vi "GridEye.vi"() -> ()   [LabVIEW 2011]
uses:
  <vilib>/gmath/interp.llb/Interpolate 2D (1d X,Y).vi
  <vilib>/gmath/NI_Gmath.lvlib
panel:
  in  "View Mode":u16(ring) items=["Back", "Front"]
  in  "temperature scaling":dbl=1.0 caption="x" format="%_4f"
  in  "?":T1(tab)
  out "Values 0":dbl[](array[numeric]) format="%.2g"
  out "Values 3":dbl[](array[numeric]) format="%.2g"
  out "Values 2":dbl[](array[numeric]) format="%.2g"
  out "Values 1":dbl[](array[numeric]) format="%.2g"
  out "Values 7":dbl[](array[numeric]) format="%.2g"
  out "Values 6":dbl[](array[numeric]) format="%.2g"
  out "Values 5":dbl[](array[numeric]) format="%.2g"
  out "Values 4":dbl[](array[numeric]) format="%.2g"
  out "temperature values":dbl[][](graph)=[[-24.0, -22.0, -20.0, -18.0, -16.0, -14.0, -12.0, -10.0], [-8.0, -6.0, -4.0, -2.0, 0.0, 2.0, 4.0, 6.0], [8.0, 10.0, 12.0, 14.0, 16.0, 18.0, 20.0, 22.0], [24.0, 26.0, 28.0, 30.0, 32.0, 34.0, 36.0, 38.0], [40.0, 42.0, 44.0, 46.0, 48.0, 50.0, 52.0, 54.0], [56.0, 58.0, 60.0, 62.0, 64.0, 66.0, 68.0, 70.0], [72.0, 74.0, 76.0, 78.0, 80.0, 82.0, 84.0, 86.0], [88.0, 90.0, 92.0, 94.0, 96.0, 98.0, 100.0, 102.0]]
  in  "Interpolation\nloops":u8(slide)=2 max=5 step=1 scale=0.0..5.0
  out "interpolated view":dbl[][](graph)=[[-24.0, -22.0, -20.0, -18.0, -16.0, -14.0, -12.0, -10.0], [-8.0, -6.0, -4.0, -2.0, 0.0, 2.0, 4.0, 6.0], [8.0, 10.0, 12.0, 14.0, 16.0, 18.0, 20.0, 22.0], [24.0, 26.0, 28.0, 30.0, 32.0, 34.0, 36.0, 38.0], [40.0, 42.0, 44.0, 46.0, 48.0, 50.0, 52.0, 54.0], [56.0, 58.0, 60.0, 62.0, 64.0, 66.0, 68.0, 70.0], [72.0, 74.0, 76.0, 78.0, 80.0, 82.0, 84.0, 86.0], [88.0, 90.0, 92.0, 94.0, 96.0, 98.0, 100.0, 102.0]]
  out "Thermistor temperature":dbl caption="°C" format="%.4g"
  in  "temperature to color scaling":enum32{"manual", "automatic"}(tab)
  in  "max":dbl=100.0 caption="°C"
  in  "min":dbl=-20.0 caption="°C"
  in  "Auto scale step size":u8=1 caption="°C"
  in  "Spread spectrum":bool
  in  "Update Speed":u16(ring) items=["10 Hz", "1 Hz"]
  in  "Output Mode":u16(ring) items=["normal", "moving average"]
  # "Enables a better visualization\nof temperature differences"
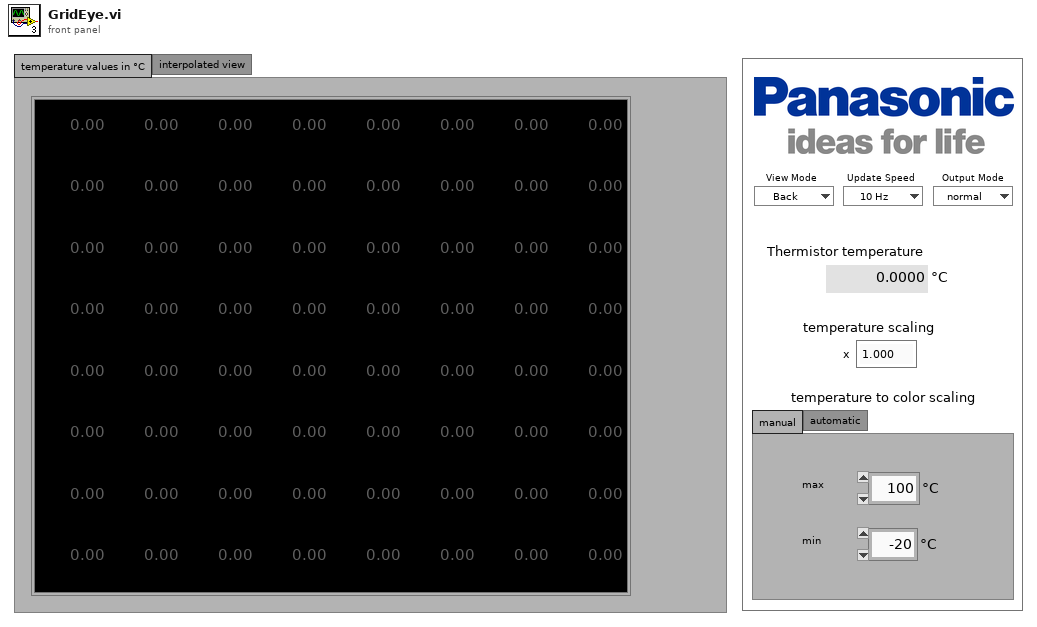
[diagram p1: front panel]
types:
  T1 = enum32{"temperature values in °C", "interpolated view"}
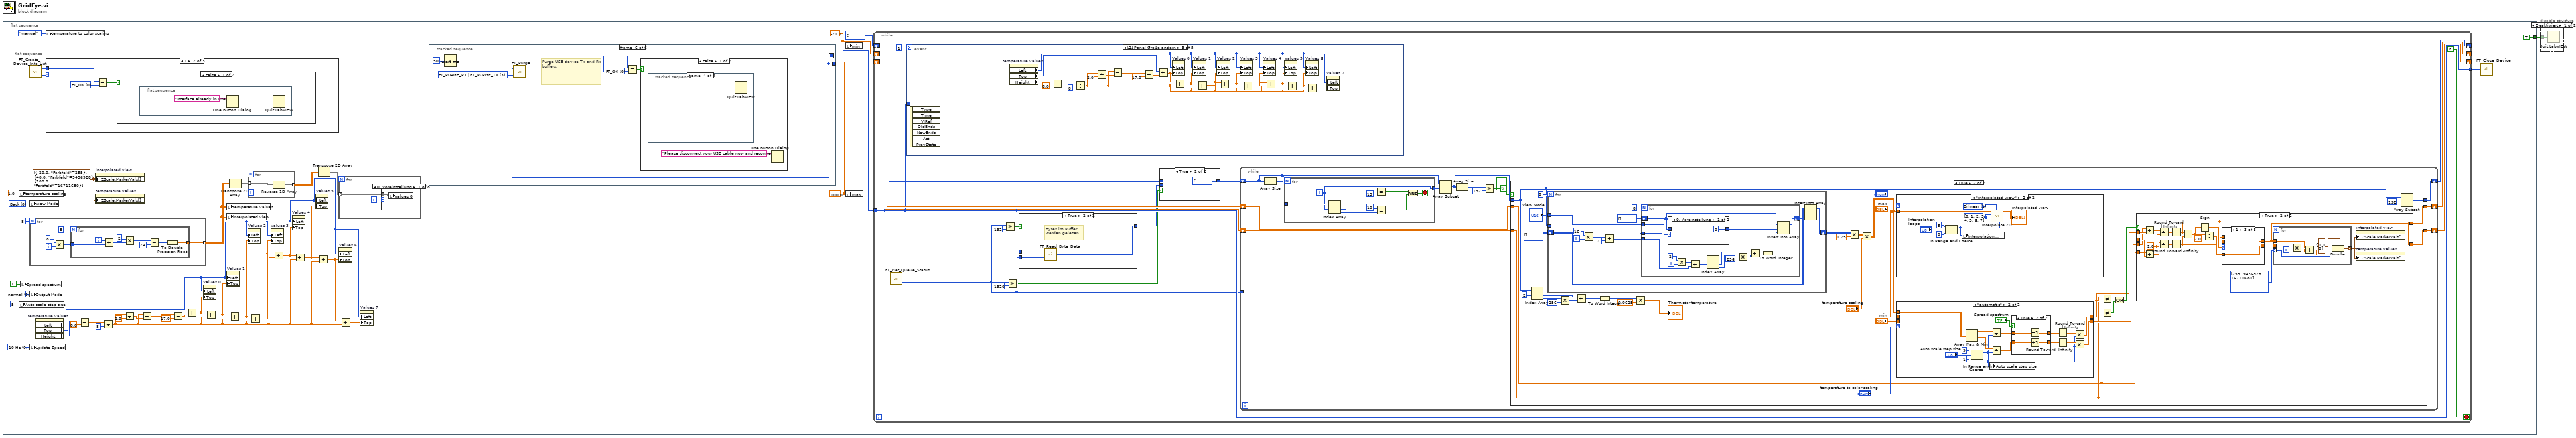
[diagram p0: block diagram]
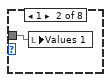
[diagram p3: hidden frame]
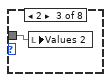
[diagram p4: hidden frame]
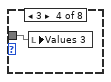
[diagram p5: hidden frame]
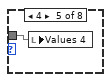
[diagram p6: hidden frame]
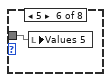
[diagram p7: hidden frame]
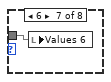
[diagram p8: hidden frame]
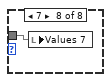
[diagram p9: hidden frame]
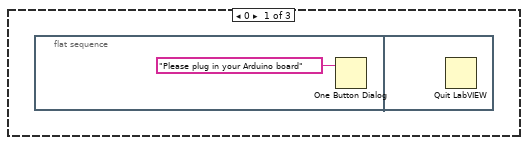
[diagram p10: hidden frame]
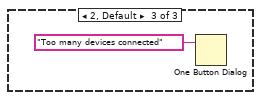
[diagram p12: hidden frame]
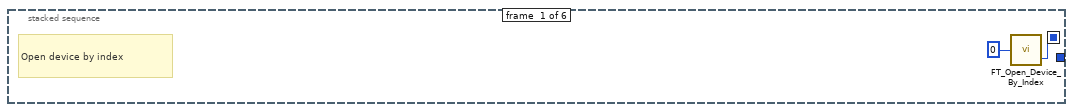
[diagram p13: hidden frame]
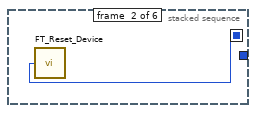
[diagram p14: hidden frame]
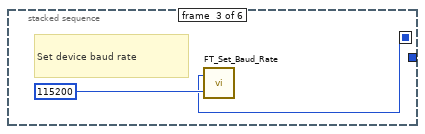
[diagram p15: hidden frame]
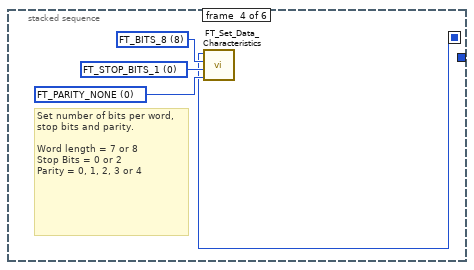
[diagram p16: hidden frame]
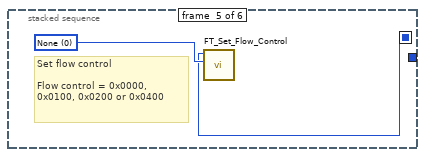
[diagram p17: hidden frame]
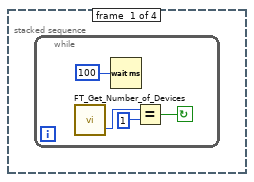
[diagram p18: hidden frame]
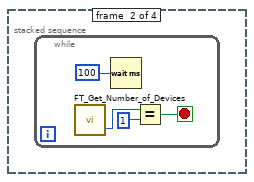
[diagram p19: hidden frame]
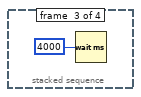
[diagram p20: hidden frame]
diagram:
  n1 = flat-sequence {
    tunnel: [TRUE ("Stopp? (T)")] -> w1
    frame #0 {
      w22 = u16 0 items=["Back", "Front"] ("View Mode")
      w25 = cluster{dbl, "Farbfeld":u32}[] [{-20.0, "Farbfeld"=255}, {40.0, "Farbfeld"=9436928}, {100.0, "Farbfeld"=16711680}] ("Array")
      w33 = u16 0 items=["normal", "moving average"] ("Output Mode")
      w34 = u16 0 items=["10 Hz", "1 Hz"] ("Update Speed")
      n2 = flat-sequence {
        frame #0 {
          n3 = call "FT_Create_Device_Info_List.vi"() -> ("Number of Devices"=w45:u32, "FT_Status"=w46:u32)
          n4 = case shown="1" w45 {
            tunnel: w46 -> [_ w50 _]
            frame 0 {
              n5 = flat-sequence {
                frame #0 {
                  n6 = One Button Dialog(message="Please plug in your Arduino board" ("Nachricht")) -> ()  [unwired: 1 in, 1 out]
                }
                frame #1 {
                  n7 = Quit LabVIEW() -> ()  [unwired: 1 in]
                }
              }
            }
            frame 1 {
              w49 = u32 0 items=["FT_OK", "FT_INVALID_HANDLE", "FT_DEVICE_NOT_FOUND", "FT_DEVICE_NOT_OPENED", "FT_IO_ERROR", "FT_INSUFFICIENT_RESOURCES", "FT_INVALID_PARAMETER", "FT_INVALID_BAUD_RATE", "FT_DEVICE_NOT_OPENED_FOR_ERASE", "FT_DEVICE_NOT_OPENED_FOR_WRITE", "FT_FAILED_TO_WRITE_DEVICE", "FT_EEPROM_READ_FAILED", "FT_EEPROM_WRITE_FAILED", "FT_EEPROM_ERASE_FAILED", "FT_EEPROM_NOT_PRESENT", "FT_EEPROM_NOT_PROGRAMMED", "FT_INVALID_ARGS", "FT_NOT_SUPPORTED", "FT_OTHER_ERROR"] ("FT_Status 4")
              n8 = Equal?(x=w50, y=w49) -> (x = y?=w48:bool)
              n9 = case shown="False" w48 {
                frame False {
                  n10 = flat-sequence {
                    frame #0 {
                      n11 = One Button Dialog(message="Interface already in use" ("Nachricht")) -> ()  [unwired: 1 in, 1 out]
                    }
                    frame #1 {
                      n12 = Quit LabVIEW() -> ()  [unwired: 1 in]
                    }
                  }
                }
                frame True {
                }
              }
            }
            frame 2, Default {
              n13 = One Button Dialog(message="Too many devices connected" ("Nachricht")) -> ()  [unwired: 1 in, 1 out]
            }
          }
        }
      }
      n14 = local write "temperature scaling"(1.0 ("temperature scaling")) -> ()
      n15 = local write "Auto scale step size"(u8 5 ("Autoscale step size")) -> ()
      n16 = local write "Spread spectrum"(TRUE ("stop")) -> ()
      n17 = local write "View Mode"(w22) -> ()
      n18 = for {
        N: 8 -> [_]
        tunnel: [w55] -> w29 mode=indexing
        i -> [w58]
        n19 = Multiply(x=8, y=w58) -> (x*y=w56:i32)
        n20 = for {
          N: 8 -> [_]
          tunnel: w56 -> [w62]
          tunnel: [w60] -> w55 mode=indexing
          i -> [w64]
          n21 = Add(x=w64, y=w62) -> (x+y=w63:i32)
          n22 = Multiply(x=2, y=w63) -> (x*y=w65:i32)
          n23 = Subtract(x=w65, y=24) -> (x-y=w61:i32)
          n24 = To Double Precision Float(number=w61) -> (double precision float=w60:dbl)
        }
      }
      n25 = local write "Output Mode"(w33) -> ()
      n26 = local write "Update Speed"(w34) -> ()
      n27 = property on="temperature values" class="IntGraph (strikt)"() -> ("Left"=w4:i32, "Top"=w3:i32, "Height"=w2:u32)  [unwired: 2 in, 2 out]
      n28 = local write "temperature to color scaling"(enum32{"manual", "automatic"}."manual" ("temperature to color scaling")) -> ()
      n29 = Subtract(x=w2, y=8.0) -> (x-y=w21:dbl)
      n30 = property on="interpolated view" class="IntGraph (strikt)"("ZScale.MarkerVals[]"=w25) -> ()  [unwired: 2 in, 2 out]
      n31 = property on="temperature values" class="IntGraph (strikt)"("ZScale.MarkerVals[]"=w25) -> ()  [unwired: 2 in, 2 out]
      n32 = Divide(x=w21, y=u32 8) -> (x/y=w19:dbl)
      n33 = Divide(x=w19, y=2.0) -> (x/y=w15:dbl)
      n34 = Subtract(x=w19, y=w15) -> (x-y=w16:dbl)
      n35 = Subtract(x=w16, y=17.0) -> (x-y=w18:dbl)
      n36 = Add(x=w3, y=w18) -> (x+y=w5:dbl)
      n37 = property on="Values 0" class="Arr (strikt)"("Left"=w4, "Top"=w5) -> ()  [unwired: 2 in, 2 out]
      n38 = Add(x=w5, y=w19) -> (x+y=w6:dbl)
      n39 = local write "temperature values"(w29) -> ()
      n40 = local write "interpolated view"(w29) -> ()
      n41 = property on="Values 1" class="Arr (strikt)"("Left"=w4, "Top"=w6) -> ()  [unwired: 2 in, 2 out]
      n42 = Add(x=w6, y=w19) -> (x+y=w7:dbl)
      n43 = Transpose 2D Array(2D array=w29) -> (transposed array=w31:dbl[][])
      n44 = for {
        tunnel: w31 -> [w54] mode=indexing
        tunnel: [w53] -> w30 mode=indexing
        n45 = Reverse 1D Array(array=w54) -> (reversed array=w53:dbl[])
      }
      n46 = property on="Values 2" class="Arr (strikt)"("Left"=w4, "Top"=w7) -> ()  [unwired: 2 in, 2 out]
      n47 = Add(x=w7, y=w19) -> (x+y=w8:dbl)
      n48 = property on="Values 3" class="Arr (strikt)"("Left"=w4, "Top"=w8) -> ()  [unwired: 2 in, 2 out]
      n49 = Add(x=w8, y=w19) -> (x+y=w9:dbl)
      n50 = property on="Values 4" class="Arr (strikt)"("Left"=w4, "Top"=w9) -> ()  [unwired: 2 in, 2 out]
      n51 = Add(x=w9, y=w19) -> (x+y=w10:dbl)
      n52 = property on="Values 5" class="Arr (strikt)"("Left"=w4, "Top"=w10) -> ()  [unwired: 2 in, 2 out]
      n53 = Add(x=w10, y=w19) -> (x+y=w11:dbl)
      n54 = Transpose 2D Array(2D array=w30) -> (transposed array=w28:dbl[][])
      n55 = for {
        tunnel: w28 -> [w35] mode=indexing
        i -> [w36]
        n56 = case shown="0, Voreinstellung" w36 {
          tunnel: w35 -> [w37 w38 w39 w40 w41 w42 w43 w44]
          frame 0, Default {
            n57 = local write "Values 0"(w37) -> ()
          }
          frame 1 {
            n58 = local write "Values 1"(w38) -> ()
          }
          frame 2 {
            n59 = local write "Values 2"(w39) -> ()
          }
          frame 3 {
            n60 = local write "Values 3"(w40) -> ()
          }
          frame 4 {
            n61 = local write "Values 4"(w41) -> ()
          }
          frame 5 {
            n62 = local write "Values 5"(w42) -> ()
          }
          frame 6 {
            n63 = local write "Values 6"(w43) -> ()
          }
          frame 7 {
            n64 = local write "Values 7"(w44) -> ()
          }
        }
      }
      n65 = property on="Values 6" class="Arr (strikt)"("Left"=w4, "Top"=w11) -> ()  [unwired: 2 in, 2 out]
      n66 = Add(x=w11, y=w19) -> (x+y=w12:dbl)
      n67 = property on="Values 7" class="Arr (strikt)"("Left"=w4, "Top"=w12) -> ()  [unwired: 2 in, 2 out]
    }
    frame #1 {
      w68 = -20.0 ("min")
      w69 = 100.0 ("max")
      n68 = stacked-sequence {
        seq-local: [w74 _ _ _ _ _] -> [_ w76 w77 w79 w83 w88]
        tunnel: [_ _ _ _ _ w88] -> w71
        frame #0 {
          # "Open device by index"
          n69 = call "FT_Open_Device_By_Index.vi"("Device Index"=u32 0) -> ("Handle"=w74:u32)  [unwired: 1 out]
        }
        frame #1 {
          n70 = call "FT_Reset_Device.vi"("Handle"=w76) -> ()  [unwired: 1 out]
        }
        frame #2 {
          # "Set device baud rate"
          n71 = call "FT_Set_Baud_Rate.vi"("Baud Rate"=u32 115200, "Handle"=w77) -> ()  [unwired: 1 out]
        }
        frame #3 {
          w81 = u8 0 items=["FT_PARITY_NONE", "FT_PARITY_ODD", "FT_PARITY_EVEN", "FT_PARITY_MARK", "FT_PARITY_SPACE"] ("Parity")
          w82 = u8 0 items=["FT_STOP_BITS_1"=0, "FT_STOP_BITS_2"=2] ("Stop Bits")
          w80 = u8 8 items=["FT_BITS_7"=7, "FT_BITS_8"=8] ("Word Length")
          # "Set number of bits per word, stop bits and parity.\n\nWord length = 7 or 8\nStop Bits = 0 or 2\nParity = 0, 1, 2, 3 or 4"
          n72 = call "FT_Set_Data_Characteristics.vi"("Parity"=w81, "Stop Bits"=w82, "Word Length"=w80, "Handle"=w79) -> ()  [unwired: 1 out]
        }
        frame #4 {
          w84 = u16 0 items=["None"=0, "RTS-CTS"=256, "DTR-DSR"=512, "XOn-XOff"=1024] ("Flow Control")
          # "Set flow control\n\nFlow control = 0x0000, 0x0100, 0x0200 or 0x0400"
          n73 = call "FT_Set_Flow_Control.vi"("Flow Control"=w84, "Handle"=w83) -> ()  [unwired: 2 in, 1 out]
        }
        frame #5 {
          w86 = u32 0 items=["FT_OK", "FT_INVALID_HANDLE", "FT_DEVICE_NOT_FOUND", "FT_DEVICE_NOT_OPENED", "FT_IO_ERROR", "FT_INSUFFICIENT_RESOURCES", "FT_INVALID_PARAMETER", "FT_INVALID_BAUD_RATE", "FT_DEVICE_NOT_OPENED_FOR_ERASE", "FT_DEVICE_NOT_OPENED_FOR_WRITE", "FT_FAILED_TO_WRITE_DEVICE", "FT_EEPROM_READ_FAILED", "FT_EEPROM_WRITE_FAILED", "FT_EEPROM_ERASE_FAILED", "FT_EEPROM_NOT_PRESENT", "FT_EEPROM_NOT_PROGRAMMED", "FT_INVALID_ARGS", "FT_NOT_SUPPORTED", "FT_OTHER_ERROR"] ("FT_Status 4")
          w90 = u32 3 items=["FT_PURGE_RX"=1, "FT_PURGE_TX"=2, "FT_PURGE_RX | FT_PURGE_TX"=3] ("Purge Flags")
          # "Purge USB device Tx and Rx  buffers."
          n74 = Wait (ms)(milliseconds to wait=u32 50 ("Zu wartende ms")) -> ()  [unwired: 1 out]
          n75 = call "FT_Purge.vi"("Purge Flags"=w90, "Handle"=w88) -> ("FT_Status"=w85:u32)
          n76 = Equal?(x=w85, y=w86) -> (x = y?=w87:bool)
          n77 = case shown="False" w87 {
            frame False {
              n78 = stacked-sequence {
                frame #0 {
                  n79 = while {
                    stop <- w94 continue-if-true
                    n80 = call "FT_Get_Number_of_Devices.vi"() -> ("Number of Devices"=w93:u16)  [unwired: 1 out]
                    n81 = Wait (ms)(milliseconds to wait=u32 100 ("Zu wartende ms")) -> ()  [unwired: 1 out]
                    n82 = Equal?(x=w93, y=u16 1) -> (x = y?=w94:bool)
                  }
                }
                frame #1 {
                  n83 = while {
                    stop <- w98 stop-if-true
                    n84 = call "FT_Get_Number_of_Devices.vi"() -> ("Number of Devices"=w97:u16)  [unwired: 1 out]
                    n85 = Wait (ms)(milliseconds to wait=u32 100 ("Zu wartende ms")) -> ()  [unwired: 1 out]
                    n86 = Equal?(x=w97, y=u16 1) -> (x = y?=w98:bool)
                  }
                }
                frame #2 {
                  n87 = Wait (ms)(milliseconds to wait=u32 4000 ("Zu wartende ms")) -> ()  [unwired: 1 out]
                }
                frame #3 {
                  n88 = Quit LabVIEW() -> ()  [unwired: 1 in]
                }
              }
              n89 = One Button Dialog(message="Please disconnect your USB cable now and reconnect it") -> ()  [unwired: 1 in, 1 out]
            }
            frame True {
            }
          }
        }
      }
      n90 = local write "min"(w68) -> ()
      n91 = local write "max"(w69) -> ()
      n92 = while {
        shift-right: [w116] -> _
        shift-left: u8[] [] -> [w104]
        tunnel: w71 -> [w110]
        tunnel: [w110] -> w70
        shift-right: [w113] -> _
        shift-left: w68 -> [w112]
        shift-right: [w109] -> _
        shift-left: w69 -> [w108]
        stop <- FALSE stop-if-true
        n93 = call "FT_Get_Queue_Status.vi"("Handle"=w110) -> ("Bytes Waiting"=w106:u32)  [unwired: 1 out]
        n94 = event shown="[2] Panel-Größe ändern" {
          selector: _ -> [_ _ _ _ _]
          dyn-events: _ -> [_ _ _ _ _]
          timeout: 1 -> [_ _ _ _ _]
          tunnel: w110 -> [_ w121 _ w147 w155]
          event Timeout {
            n95 = event-data() -> ()  [unwired: 1 in, 2 out]
          }
          event "Update Speed": Value Change {
            n96 = event-data() -> ("NewVal"=w125:u16)  [unwired: 1 in, 4 out]
            n97 = Build Array(u16 2 ("NeuerWert"), w125) -> (w122:u16[])
            n98 = Array Size(array=w122) -> (size(s)=w124:i32)
            n99 = To Unsigned Long Integer(number=w124) -> (unsigned 32bit integer=w123:u32)
            n100 = call "FT_Write_Byte_Data.vi"("Bytes To Write"=w123, "Buffer"=w122, "Handle"=w121) -> ()  [unwired: 2 out]
          }
          event Panel Resize {
            n101 = event-data() -> ()  [unwired: 1 in, 7 out]
            n102 = property on="temperature values" class="IntGraph (strikt)"() -> ("Left"=w133:i32, "Top"=w140:i32, "Height"=w128:u32)  [unwired: 2 in, 2 out]
            n103 = Subtract(x=w128, y=8.0) -> (x-y=w127:dbl)
            n104 = Divide(x=w127, y=u32 8) -> (x/y=w131:dbl)
            n105 = Divide(x=w131, y=2.0) -> (x/y=w144:dbl)
            n106 = Subtract(x=w131, y=w144) -> (x-y=w143:dbl)
            n107 = Subtract(x=w143, y=17.0) -> (x-y=w141:dbl)
            n108 = Add(x=w140, y=w141) -> (x+y=w139:dbl)
            n109 = property on="Values 0" class="Arr (strikt)"("Left"=w133, "Top"=w139) -> ()  [unwired: 2 in, 2 out]
            n110 = Add(x=w139, y=w131) -> (x+y=w138:dbl)
            n111 = property on="Values 1" class="Arr (strikt)"("Left"=w133, "Top"=w138) -> ()  [unwired: 2 in, 2 out]
            n112 = Add(x=w138, y=w131) -> (x+y=w137:dbl)
            n113 = property on="Values 2" class="Arr (strikt)"("Left"=w133, "Top"=w137) -> ()  [unwired: 2 in, 2 out]
            n114 = Add(x=w137, y=w131) -> (x+y=w136:dbl)
            n115 = property on="Values 3" class="Arr (strikt)"("Left"=w133, "Top"=w136) -> ()  [unwired: 2 in, 2 out]
            n116 = Add(x=w136, y=w131) -> (x+y=w135:dbl)
            n117 = property on="Values 4" class="Arr (strikt)"("Left"=w133, "Top"=w135) -> ()  [unwired: 2 in, 2 out]
            n118 = Add(x=w135, y=w131) -> (x+y=w134:dbl)
            n119 = property on="Values 5" class="Arr (strikt)"("Left"=w133, "Top"=w134) -> ()  [unwired: 2 in, 2 out]
            n120 = Add(x=w134, y=w131) -> (x+y=w132:dbl)
            n121 = property on="Values 6" class="Arr (strikt)"("Left"=w133, "Top"=w132) -> ()  [unwired: 2 in, 2 out]
            n122 = Add(x=w132, y=w131) -> (x+y=w130:dbl)
            n123 = property on="Values 7" class="Arr (strikt)"("Left"=w133, "Top"=w130) -> ()  [unwired: 2 in, 2 out]
          }
          event "Output Mode": Value Change {
            n124 = event-data() -> ("NewVal"=w153:u16)  [unwired: 1 in, 4 out]
            n125 = Scale By Power Of 2(n=5, x=w153) -> (x*2^n=w151:u16)
            n126 = Build Array(u16 7 ("NeuerWert"), w151) -> (w148:u16[])
            n127 = Array Size(array=w148) -> (size(s)=w150:i32)
            n128 = To Unsigned Long Integer(number=w150) -> (unsigned 32bit integer=w149:u32)
            n129 = call "FT_Write_Byte_Data.vi"("Bytes To Write"=w149, "Buffer"=w148, "Handle"=w147) -> ()  [unwired: 2 out]
          }
          event Application Instance Close? {
            n130 = event-data() -> ("SilentShutdown"=w156:bool)  [unwired: 1 in, 3 out]
            n131 = call "FT_Close_Device.vi"("Handle"=w155) -> ()  [unwired: 1 out]
            n132 = event-data("SilentShutdown"=w156) -> ()  [unwired: 2 in, 1 out]
          }
        }
        n133 = Greater Or Equal?(x=w106, y=u32 132) -> (x >= y?=w114:bool)
        n134 = Greater Or Equal?(x=w106, y=u32 1320) -> (x >= y?=w105:bool)
        n135 = case shown="True" w114 {
          tunnel: [u8[] [] ("Read Data") w160] -> w102
          tunnel: w110 -> [_ w158]
          tunnel: w106 -> [_ w159]
          frame False {
          }
          frame True {
            # "Bytes im Puffer werden gelesen."
            n136 = call "FT_Read_Byte_Data.vi"("Handle"=w158, "Bytes To Read"=w159) -> ("Read Data"=w160:u8[])  [unwired: 2 out]
          }
        }
        n137 = case shown="True" w105 {
          tunnel: w104 -> [w119 _]
          tunnel: [w118 u8[] []] -> w103
          tunnel: w102 -> [w117 _]
          frame False {
            n138 = Insert Into Array(array=w119, new element=w117) -> (w118:u8[])  [unwired: 1 in]
          }
          frame True {
          }
        }
        n139 = while {
          shift-right: [w166] -> w116
          shift-left: w103 -> [w172]
          tunnel: w106 -> [_]
          shift-right: [w164] -> w113
          shift-left: w112 -> [w163]
          shift-right: [w162] -> w109
          shift-left: w108 -> [w161]
          stop <- w167 continue-if-true
          n140 = Array Size(array=w172) -> (size(s)=w171:i32)
          n141 = for {
            N: w171 -> [_]
            tunnel: w172 -> [w327]
            tunnel: [w325] -> w165
            i -> [w325]
            stop <- w326 stop-if-true
            n142 = Index Array(array=w327, index #1=w325) -> (element #1=w328:u8, element #2=w330:u8)  [unwired: 1 in]
            n143 = Equal?(x=w328, y=u8 13) -> (x = y?=w331:bool)
            n144 = Equal?(x=u8 10 ("y"), y=w330) -> (x = y?=w332:bool)
            n145 = And(x=w331, y=w332) -> (x .and. y?=w326:bool)
          }
          n146 = Array Subset(array=w172, index=w165) -> (w168:u8[])  [unwired: 1 in]
          n147 = Array Size(array=w168) -> (size(s)=w170:i32)
          n148 = Greater Or Equal?(x=w170, y=132) -> (x >= y?=w167:bool)
          n149 = case shown="True" w167 {
            tunnel: w168 -> [w175 w192]
            tunnel: [w175 w206] -> w166
            tunnel: [w174 w183] -> w164
            tunnel: w163 -> [w174 w185]
            tunnel: [w173 w182] -> w162
            tunnel: w161 -> [w173 w184]
            frame False {
            }
            frame True {
              n150 = Index Array(array=w192, index #1=2 ("Index")) -> (element #1=w199:u8, element #2=w200:u8)  [unwired: 1 in]
              n151 = for {
                N: 8 -> [_]
                tunnel: w192 -> [w304]
                shift-right: [w295] -> w178
                shift-left: i16[][] [] -> [w297]
                tunnel: "View Mode" -> [w294]
                i -> [w302]
                n152 = Multiply(x=16, y=w302) -> (x*y=w301:i32)
                n153 = Add(x=w301, y=4) -> (x+y=w300:i32)
                n154 = for {
                  N: 8 -> [_]
                  tunnel: w304 -> [w321]
                  tunnel: w300 -> [w316]
                  shift-right: [w310] -> w296
                  shift-left: i16[] [] -> [w306]
                  tunnel: w294 -> [w307]
                  i -> [w320]
                  n155 = case shown="0, Voreinstellung" w307 {
                    tunnel: [0 ("Index") w323] -> w309
                    tunnel: w306 -> [_ w324]
                    frame 0, Default {
                    }
                    frame 1 {
                      n156 = Array Size(array=w324) -> (size(s)=w323:i32)
                    }
                  }
                  n157 = Multiply(x=2, y=w320) -> (x*y=w317:i32)
                  n158 = Add(x=w317, y=w316) -> (x+y=w315:i32)
                  n159 = Index Array(array=w321, index #1=w315) -> (element #1=w313:u8, element #2=w312:u8)  [unwired: 1 in]
                  n160 = Multiply(x=w312, y=u16 256) -> (x*y=w311:u16)
                  n161 = Add(x=w313, y=w311) -> (x+y=w314:u16)
                  n162 = To Word Integer(number=w314) -> (16bit integer=w308:i16)
                  n163 = Insert Into Array(array=w306, index=w309, new element=w308) -> (w310:i16[])
                }
                n164 = Insert Into Array(array=w297, new element=w296) -> (w295:i16[][])  [unwired: 2 in]
              }
              n165 = Multiply(x=w200, y=i16 256) -> (x*y=w201:i16)
              n166 = Add(x=w199, y=w201) -> (x+y=w198:i16)
              n167 = To Word Integer(number=w198) -> (16bit integer=w195:i16)
              n168 = Multiply(x=w195, y=0.0625 ("x")) -> (x*y=→"Thermistor temperature":dbl)
              n169 = Multiply(x=w178, y=0.25 ("x")) -> (x*y=w181:dbl[][])
              n170 = Multiply(x=w181, y="temperature scaling") -> (x*y=w179:dbl[][])
              n171 = case shown="\"interpolated view\"" "?" {
                tunnel: w179 -> [w271 w288]
                frame "temperature values in °C", Default {
                  n172 = Transpose 2D Array(2D array=w271) -> (transposed array=w272:dbl[][])
                  n173 = for {
                    tunnel: w272 -> [w285] mode=indexing
                    tunnel: [w284] -> w273 mode=indexing
                    n174 = Reverse 1D Array(array=w285) -> (reversed array=w284:dbl[])
                  }
                  n175 = Transpose 2D Array(2D array=w273) -> (transposed array=w270:dbl[][])
                  n176 = for {
                    tunnel: w270 -> [w274] mode=indexing
                    i -> [w275]
                    n177 = case shown="0, Voreinstellung" w275 {
                      tunnel: w274 -> [w276 w277 w278 w279 w280 w281 w282 w283]
                      frame 0, Default {
                        "Values 0" <- w276
                      }
                      frame 1 {
                        "Values 1" <- w277
                      }
                      frame 2 {
                        "Values 2" <- w278
                      }
                      frame 3 {
                        "Values 3" <- w279
                      }
                      frame 4 {
                        "Values 4" <- w280
                      }
                      frame 5 {
                        "Values 5" <- w281
                      }
                      frame 6 {
                        "Values 6" <- w282
                      }
                      frame 7 {
                        "Values 7" <- w283
                      }
                    }
                  }
                  "temperature values" <- w271
                }
                frame "interpolated view" {
                  w290 = i32[] [0, 1, 2, 3, 4, 5, 6, 7] ("Array")
                  w291 = 1 items=["Nächste", "Bilinear", "Bikubisch", "Spline (bikubisch)"] ("method")
                  n178 = In Range and Coerce(upper limit=u8 5 ("Obergrenze"), x="Interpolation\nloops", lower limit=u8 0 ("Untergrenze")) -> (coerced(x)=w289:u8)  [unwired: 1 out]
                  n179 = local write "Interpolation\nloops"(w289) -> ()
                  n180 = call-poly <vilib>:"Interpolate 2D.vi"("ntimes"=w289, "method"=w291, "Y"=w290, "X"=w290, "Z"=w288) -> ("zi"=→"interpolated view":dbl[][])  [unwired: 3 in, 3 out]
                }
              }
              n181 = case shown="\"automatic\"" "temperature to color scaling" {
                tunnel: w179 -> [_ w263]
                tunnel: "min" -> [w246 _]
                tunnel: "max" -> [w247 _]
                tunnel: [w247 w256] -> w187
                tunnel: [w246 w253] -> w186
                frame "manual", Default {
                }
                frame "automatic" {
                  n182 = Array Max & Min(array=w263) -> (max value=w258:dbl, min value=w259:dbl)  [unwired: 2 out]
                  n183 = In Range and Coerce(upper limit=u8 9 ("Obergrenze"), x="Auto scale step size", lower limit=u8 1 ("Untergrenze")) -> (coerced(x)=w254:u8)  [unwired: 1 out]
                  n184 = local write "Auto scale step size"(w254) -> ()
                  n185 = Divide(x=w258, y=w254) -> (x/y=w252:dbl)
                  n186 = Divide(x=w259, y=w254) -> (x/y=w250:dbl)
                  n187 = case shown="True" "Spread spectrum" {
                    tunnel: w250 -> [w265 w267]
                    tunnel: w252 -> [w264 w269]
                    tunnel: [w264 w268] -> w251
                    tunnel: [w265 w266] -> w249
                    frame False {
                    }
                    frame True {
                      n188 = Decrement(x=w269) -> (x-1=w268:dbl)
                      n189 = Increment(x=w267) -> (x+1=w266:dbl)
                    }
                  }
                  n190 = Round Toward +Infinity(x=w251) -> (ceil(x): smallest int >= x=w257:dbl)
                  n191 = Round Toward -Infinity(1:w249) -> (0:w255:dbl)
                  n192 = Multiply(x=w257, y=w254) -> (x*y=w256:dbl)
                  n193 = Multiply(x=w255, y=w254) -> (x*y=w253:dbl)
                }
              }
              n194 = Not Equal?(x=w184, y=w187) -> (x != y?=w189:bool)
              n195 = Not Equal?(x=w186, y=w185) -> (x != y?=w190:bool)
              n196 = Or(x=w189, y=w190) -> (x .or. y?=w188:bool)
              n197 = case shown="True" w188 {
                tunnel: w187 -> [_ w224]
                tunnel: w186 -> [w210 w226]
                tunnel: w185 -> [_ w219]
                tunnel: w184 -> [w209 w220]
                tunnel: [w210 w213] -> w183
                tunnel: [w209 w211] -> w182
                frame False {
                }
                frame True {
                  w218 = 2.0 ("x+1")
                  n198 = Add(x=w220, y=w224) -> (x+y=w223:dbl)
                  n199 = Add(x=w219, y=w226) -> (x+y=w225:dbl)
                  n200 = Divide(x=w223, y=w218) -> (x/y=w221:dbl)
                  n201 = Divide(x=w225, y=w218) -> (x/y=w222:dbl)
                  n202 = Round Toward +Infinity(x=w221) -> (ceil(x): smallest int >= x=w211:dbl)
                  n203 = Round Toward -Infinity(1:w222) -> (0:w212:dbl)
                  n204 = Subtract(x=w211, y=w212) -> (x-y=w217:dbl)
                  n205 = Sign(1:w217) -> (0:w216:dbl)
                  n206 = Divide(x=w217, y=2.0) -> (x/y=w215:dbl)
                  n207 = case shown="1" w216 {
                    tunnel: [w231 1.0 w237] -> w214
                    tunnel: w215 -> [w232 _ w237]
                    tunnel: [w230 w233 w236] -> w213
                    tunnel: w212 -> [_ w234 w236]
                    tunnel: w211 -> [w230 _ _]
                    frame -1 {
                      n208 = Absolute Value(x=w232) -> (abs(x)=w231:dbl)
                    }
                    frame 0, Default {
                      n209 = Decrement(x=w234) -> (x-1=w233:dbl)
                    }
                    frame 1 {
                    }
                  }
                  n210 = for {
                    tunnel: w214 -> [w244]
                    tunnel: u32[] [255, 9436928, 16711680] -> [w241] mode=indexing
                    tunnel: [w240] -> w228 mode=indexing
                    tunnel: w213 -> [w238]
                    i -> [w245]
                    n211 = Multiply(x=w244, y=w245) -> (x*y=w243:dbl)
                    n212 = Add(x=w243, y=w238) -> (x+y=w242:dbl)
                    n213 = Bundle(cluster=cluster{dbl, "Farbfeld":u32} {0.0, "Farbfeld"=0}, w242, "Farbfeld"=w241) -> (w240:cluster{dbl, "Farbfeld":u32})
                  }
                  n214 = property on="interpolated view" class="IntGraph (strikt)"("ZScale.MarkerVals[]"=w228) -> ()  [unwired: 2 in, 2 out]
                  n215 = property on="temperature values" class="IntGraph (strikt)"("ZScale.MarkerVals[]"=w228) -> ()  [unwired: 2 in, 2 out]
                }
              }
              n216 = Array Subset(array=w192, index=132 ("Index")) -> (w206:u8[])  [unwired: 1 in]
            }
          }
        }
      }
      n217 = call "FT_Close_Device.vi"("Handle"=w70) -> ()  [unwired: 1 out]
    }
  }
  n218 = disable-structure shown="Deaktiviert" {
    disable-tunnel: w1 -> [w334 _]
    frame Disabled {
      n219 = Quit LabVIEW(quit? (T)=w334) -> ()
    }
    frame Enabled {
    }
  }
